vi "Flatten.vi"(8 "error in (no error)":errorcluster, 11 "Msg in":refnum<class "Msg.lvclass">) -> (0 "error out":errorcluster, 2 "Buffer":u8[](array[numeric]) format="%.0x", 3 "Msg out":refnum<class "Msg.lvclass">)   [LabVIEW 2020, in "PB Msg Template.lvlib" / "Msg.lvclass"]
uses:
  Msg.lvclass
  PB Msg Template.lvlib
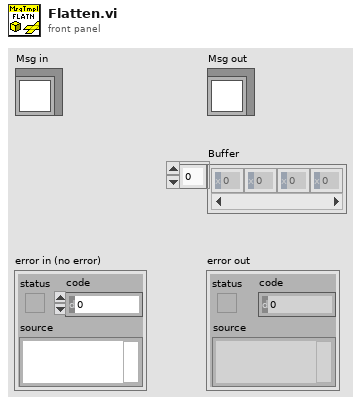
[diagram p1: front panel]
types:
  T1 = typedef "PB Msg Template.lvlib/Data.ctl" = cluster{"Numeric":dbl}
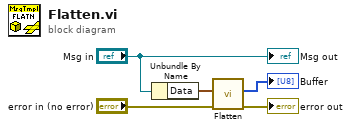
[diagram p0: block diagram]
diagram:
  n1 = Unbundle By Name("Msg in") -> ("Data"=w4:T1)
  n2 = call "Flatten.vi"("error in"="error in (no error)", 10:w4) -> ("error out"=→"error out":errorcluster, "Buffer"=→"Buffer":u8[])  [unwired: 8 in]
  "Msg out" <- "Msg in"
